vi "Project - Memory.vi"(5 "Memory":T1, 7 "Msg Chain":string, 8 "error in (no error)":errorcluster {"code" format="Error %.0f"}, 10 "Project Doc":refnum<class "Project Documentation.lvclass">, 11 "VIDoc Printer - Confluence In":refnum<class "VIDoc Printer - Confluence.lvclass">) -> (0 "error out":errorcluster {"code" format="Error %.0f"}, 3 "VIDoc Printer - Confluence Out":refnum<class "VIDoc Printer - Confluence.lvclass">)   [LabVIEW 2023, in "VIDoc Printer - Confluence.lvlib" / "VIDoc Printer - Confluence.lvclass"]
uses:
  VIDoc Printer - Confluence.lvclass
  Parsing/Project Documentation/Project Documentation.lvclass
  Parsing/TypeDefs/Memory Size Cluster.ctl
  Confluence Formatting/Types/Format Combo Box.ctl
  VIDoc Printer - Confluence.lvclass/VIDoc Printer - Confluence.ctl
  Confluence Formatting/Confluence Formatting.lvlib
  Parsing/VIDoc Parsing.lvlib
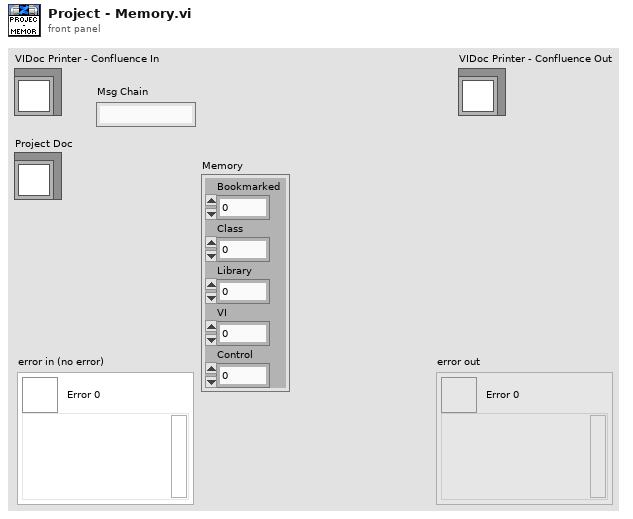
[diagram p1: front panel]
types:
  T1 = typedef "VIDoc Parsing.lvlib/Memory Size Cluster.ctl" = cluster{"Bookmarked":dbl, "Class":dbl, "Library":dbl, "VI":dbl, "Control":dbl}
  T2 = typedef "Confluence Formatting.lvlib/Format Combo Box.ctl" = string
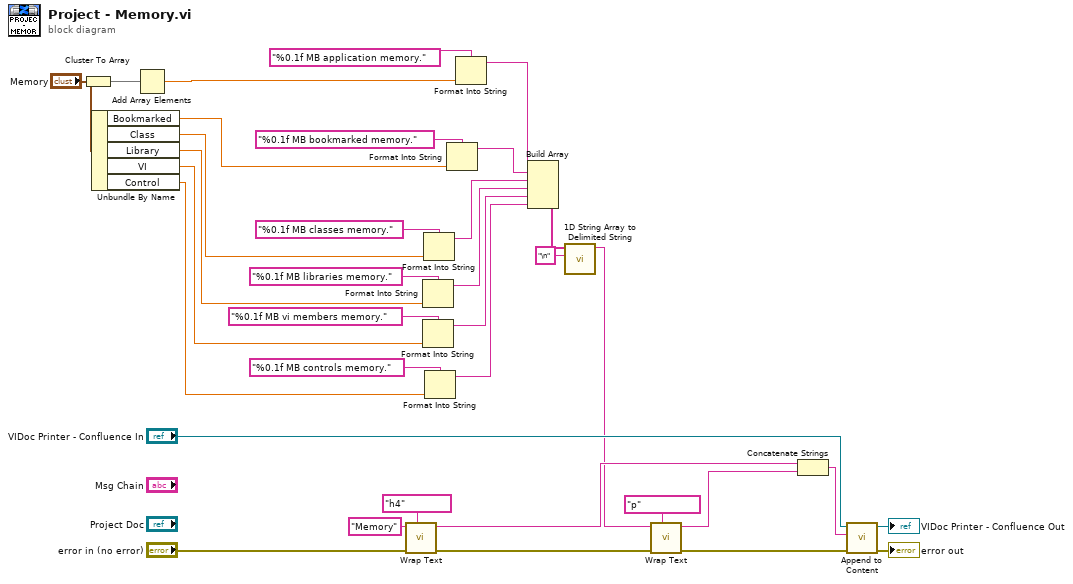
[diagram p0: block diagram]
diagram:
  n1 = Cluster To Array(cluster="Memory") -> (array=w22:dbl[])
  n2 = Unbundle By Name("Memory") -> ("Bookmarked"=w1:dbl, "Class"=w15:dbl, "Library"=w14:dbl, "VI"=w13:dbl, "Control"=w12:dbl)
  n3 = Add Array Elements(numeric array=w22) -> (sum=w21:dbl)
  n4 = call "Wrap Text.vi"("Formatting"=T2 "h4", "Error in"="error in (no error)", "String"="Memory") -> ("Error out"=w30:errorcluster, "Wrapped String"=w32:string)  [unwired: 7 in]
  n5 = Format Into String(format string="%0.1f MB libraries memory.", w14) -> (resulting string=w8:string)  [unwired: 2 in, 1 out]
  n6 = Format Into String(format string="%0.1f MB vi members memory.", w13) -> (resulting string=w7:string)  [unwired: 2 in, 1 out]
  n7 = Format Into String(format string="%0.1f MB classes memory.", w15) -> (resulting string=w9:string)  [unwired: 2 in, 1 out]
  n8 = Format Into String(format string="%0.1f MB controls memory.", w12) -> (resulting string=w6:string)  [unwired: 2 in, 1 out]
  n9 = Format Into String(format string="%0.1f MB bookmarked memory.", w1) -> (resulting string=w10:string)  [unwired: 2 in, 1 out]
  n10 = Format Into String(format string="%0.1f MB application memory.", w21) -> (resulting string=w11:string)  [unwired: 2 in, 1 out]
  n11 = Build Array(w11, w10, w9, w8, w7, w6) -> (w5:string[])
  n12 = call <vilib>:"1D String Array to Delimited String.vi"("delimiter"="\n", "string array"=w5) -> ("delimited string"=w2:string)  [unwired: 9 in]
  n13 = call "Wrap Text.vi"("Formatting"=T2 "p", "Error in"=w30, "String"=w2) -> ("Error out"=w29:errorcluster, "Wrapped String"=w31:string)  [unwired: 7 in]
  n14 = Concatenate Strings(w32, w31) -> (w28:string)
  n15 = call "Append to Content.vi"("error in (no error)"=w29, "Content"=w28, "VIDoc Printer - Confluence In"="VIDoc Printer - Confluence In") -> ("error out"=→"error out":errorcluster, "VIDoc Printer - Confluence Out"=→"VIDoc Printer - Confluence Out":refnum<class "VIDoc Printer - Confluence.lvclass">)  [unwired: 7 in]
